vi "ATF-Pump-CDT FGV.vi"(8 "error in (no error)":errorcluster, 10 "CDT":dbl, 11 "Write/Read":enum16{"Write", "Read"}(ring)) -> (0 "error Out":errorcluster, 2 "CDT Out":dbl)   [LabVIEW 2022 SP3]
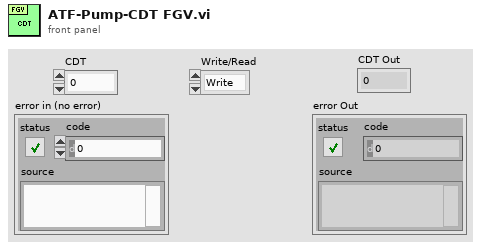
[diagram p1: front panel]
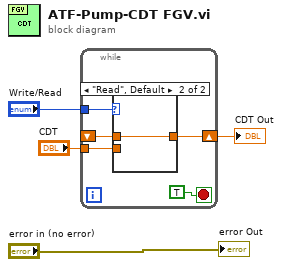
[diagram p0: block diagram]
diagram:
  n1 = while {
    shift-right: [w7] -> w3
    shift-left: _ -> [w6]
    tunnel: "CDT" -> [w8]
    tunnel: "Write/Read" -> [w5]
    stop <- TRUE stop-if-true
    n2 = case shown="\"Read\", Default" w5 {
      tunnel: w8 -> [w10 _]
      tunnel: [w10 w11] -> w7
      tunnel: w6 -> [_ w11]
      frame "Write" {
      }
      frame "Read", Default {
      }
    }
  }
  "CDT Out" <- w3
  "error Out" <- "error in (no error)"
